vi "Test TCRS Temperature At Initial Value if Heater Disabled.vi"(8 "error in (no error)":errorcluster, 11 "Thermal Chamber Response Simlator Test In":refnum<class "Thermal Chamber Response Simlator Test.lvclass">) -> (0 "error out":errorcluster, 3 "Thermal Chamber Response Simlator Test Out":refnum<class "Thermal Chamber Response Simlator Test.lvclass">)   [LabVIEW 2020, in "Thermal Chamber Response Simlator Test.lvclass"]
uses:
  Thermal Chamber Response Simlator Test.lvclass
  C:/Program Files (x86)/National Instruments/LabVIEW 2020/vi.lib/Astemes/LUnit/Test Case.lvclass
  Thermal Chamber Response Simlator/Thermal Chamber Response Simlator.lvclass
  Thermal Chamber Response Simlator/Thermal Chamber Response Simlator.lvclass/Thermal Chamber Response Simlator.ctl
  <vilib>/Astemes/LUnit/Test Case.lvclass/Test Case.ctl
  6fbb51b6-38fb-4c54-9d91-15f5180ad069.vi
  <vilib>/Astemes/LUnit/Core/LUnit Test Case/Private/Append Pass Result.vi
  <vilib>/Astemes/LUnit/Core/LUnit Test Case/Private/Append Fail Result.vi
  6fbb51b6-38fb-4c54-9d91-15f5180ad069.vi/9c5d11cd-9439-4240-a1ee-d9baace9c924.vi
  <vilib>/Astemes/LUnit/Core/LUnit Test Case/Private/Run In UI.vi
  <vilib>/Utility/error.llb/Clear Errors.vi
  Thermal Chamber Response Simlator/Private/Get Current Time if Not Set.vi
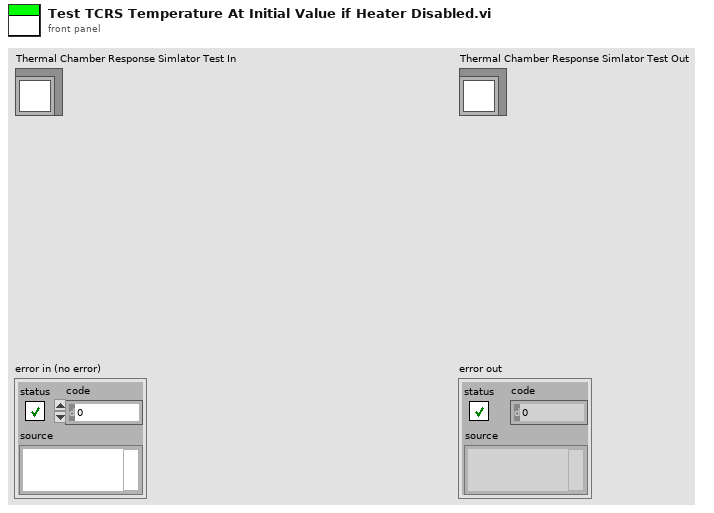
[diagram p1: front panel]
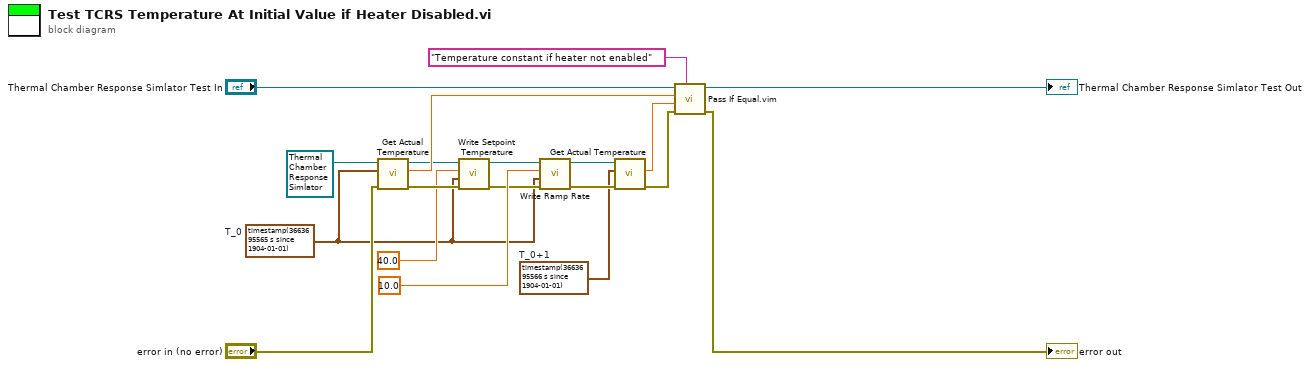
[diagram p0: block diagram]
diagram:
  w13 = timestamp(3663695566 s since 1904-01-01)  # T_0+1
  w1 = timestamp(3663695565 s since 1904-01-01)  # T_0
  n1 = call "Get Actual Temperature.vi"("error in (no error)"="error in (no error)", "Time Stamp"=w1, "Thermal Chamber Response Simlator In"=refnum<class "Thermal Chamber Response Simlator.lvclass"> refnum ("Thermal Chamber Response Simlator.lvclass")) -> ("error out"=w17:errorcluster, "Actual Temperature [degC]"=w9:dbl, "Thermal Chamber Response Simlator Out"=w4:refnum<class "Thermal Chamber Response Simlator.lvclass">)  [unwired: 6 in]
  n2 = call "Write Setpoint Temperature.vi"("error in (no error)"=w17, "Update Time"=w1, "Setpoint Temperature [degC]"=40.0, "Thermal Chamber Response Simlator In"=w4) -> ("error out"=w5:errorcluster, "Thermal Chamber Response Simlator Out"=w3:refnum<class "Thermal Chamber Response Simlator.lvclass">)  [unwired: 6 in]
  n3 = call "Write Ramp Rate.vi"("error in (no error)"=w5, "Time Stamp"=w1, "Ramp Rate [degC/s]"=10.0, "Thermal Chamber Response Simlator In"=w3) -> ("error out"=w14:errorcluster, "Thermal Chamber Response Simlator Out"=w15:refnum<class "Thermal Chamber Response Simlator.lvclass">)  [unwired: 6 in]
  n4 = call "Get Actual Temperature.vi"("error in (no error)"=w14, "Time Stamp"=w13, "Thermal Chamber Response Simlator In"=w15) -> ("error out"=w11:errorcluster, "Actual Temperature [degC]"=w10:dbl)  [unwired: 6 in, 1 out]
  n5 = call "Pass If Equal.vim"("Description"="Temperature constant if heater not enabled", "error in (no error)"=w11, "Actual"=w10, "Expected"=w9, "LUnit Test Case In"="Thermal Chamber Response Simlator Test In") -> ("error out"=→"error out":errorcluster, "LUnit Test Case Out"=→"Thermal Chamber Response Simlator Test Out":refnum<class "Thermal Chamber Response Simlator Test.lvclass">)  [unwired: 5 in]
